vi "ApplyTableAppearance_benchmarking.vi"(6 "Defer Updates? (T)":bool=TRUE, 7 "Layout Ring Ref":refnum<vi>, 8 "error in (no error)":errorcluster, 9 "Mode Index":i32=2, 10 "Col Array in":refnum<class "Column.lvclass">[](array[class]), 11 "Table Ref in":refnum<vi>) -> (0 "error out":errorcluster, 3 "Table Ref out":refnum<vi>)   [LabVIEW 2013]
doc: "(Re)Initialize table appearance from column (appearance) array. A layout reference is required so that the existing layout view is preserved. The user can choose not to 'defer panel updates,' although the default is recommended to keep the program responsive.\n\nThis VI is read-only w.r.t. the column array."
uses:
  ColumnVIs/Column/Column.lvclass
  <vilib>/Utility/miscctls.llb/LVRowAndColumnTypeDef.ctl
  Globals/StdRowHeightGlobal.vi
panel:
  out "UnDefer (ms)":u32
  out "Layout (ms)":u32
  out "Rows + Mode (ms)":u32
  out "InitAppear (ms)":u32
  out "Reset Table (ms)":u32
  out "Defer (ms)":u32
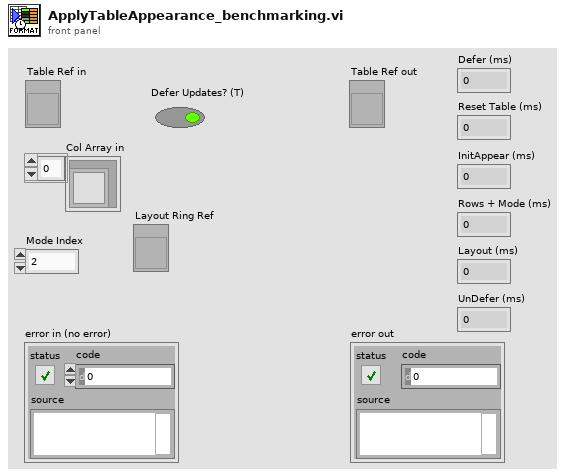
[diagram p1: front panel]
types:
  T1 = typedef "LVRowAndColumnTypeDef.ctl" = cluster{"Row":i32, "Column":i32}
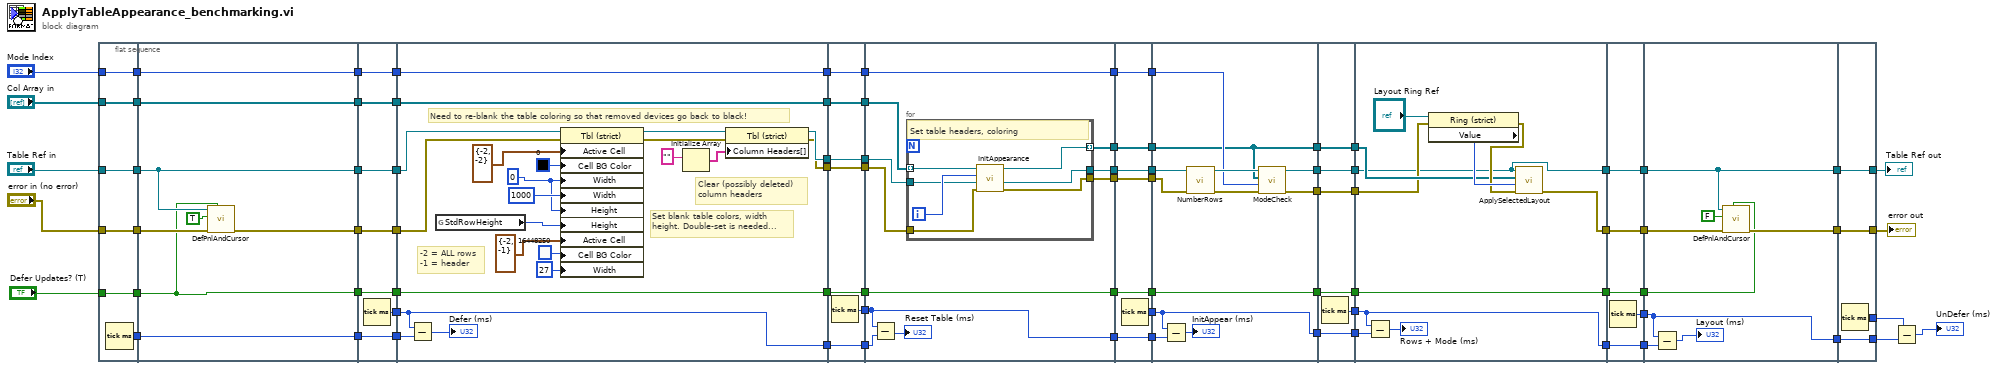
[diagram p0: block diagram]
diagram:
  n1 = flat-sequence {
    tunnel: "Mode Index" -> [w80]
    tunnel: "Col Array in" -> [w81]
    tunnel: "Table Ref in" -> [w82]
    tunnel: "Defer Updates? (T)" -> [w83]
    tunnel: "error in (no error)" -> [w84]
    tunnel: [w84] -> w70
    tunnel: [w83] -> w69
    tunnel: [w82] -> w68
    tunnel: [w81] -> w67
    tunnel: [w80] -> w66
    tunnel: [w79] -> w53
    tunnel: [w88] -> w65
    tunnel: [w87] -> w63
    tunnel: [w92] -> w61
    tunnel: [w91] -> w59
    tunnel: [w86] -> w57
    tunnel: w70 -> [w89]
    tunnel: w69 -> [w86]
    tunnel: w68 -> [w87]
    tunnel: w67 -> [w92]
    tunnel: w66 -> [w91]
    tunnel: [w90] -> w54
    tunnel: w53 -> [w90]
    tunnel: w65 -> [w99]
    tunnel: [w99] -> w64
    tunnel: w63 -> [w98]
    tunnel: [w98] -> w62
    tunnel: w61 -> [w97]
    tunnel: [w97] -> w60
    tunnel: w59 -> [w96]
    tunnel: [w96] -> w58
    tunnel: w57 -> [w95]
    tunnel: [w95] -> w56
    tunnel: [w94] -> w55
    tunnel: w54 -> [w94]
    tunnel: [w93] -> w52
    tunnel: w64 -> [w110]
    tunnel: w62 -> [w109]
    tunnel: w60 -> [w121]
    tunnel: w58 -> [w120]
    tunnel: [w111] -> w51
    tunnel: [w121] -> w49
    tunnel: [w120] -> w47
    tunnel: [w112] -> w45
    tunnel: w56 -> [w112]
    tunnel: [w108] -> w43
    tunnel: w55 -> [w106]
    tunnel: w52 -> [w105]
    tunnel: [w105] -> w40
    tunnel: w51 -> [w128]
    tunnel: [w128] -> w50
    tunnel: w49 -> [w127]
    tunnel: [w127] -> w48
    tunnel: w47 -> [w126]
    tunnel: [w126] -> w46
    tunnel: w45 -> [w125]
    tunnel: [w125] -> w44
    tunnel: w43 -> [w124]
    tunnel: [w124] -> w42
    tunnel: [w123] -> w41
    tunnel: w40 -> [w123]
    tunnel: [w122] -> w39
    tunnel: w50 -> [w133]
    tunnel: w48 -> [w138]
    tunnel: w46 -> [w139]
    tunnel: [w135] -> w38
    tunnel: [w139] -> w36
    tunnel: [w137] -> w34
    tunnel: [w136] -> w32
    tunnel: w44 -> [w136]
    tunnel: [w134] -> w30
    tunnel: w42 -> [w132]
    tunnel: w41 -> [w130]
    tunnel: w39 -> [w129]
    tunnel: [w129] -> w27
    tunnel: w38 -> [w153]
    tunnel: [w153] -> w37
    tunnel: w36 -> [w152]
    tunnel: [w152] -> w35
    tunnel: w34 -> [w151]
    tunnel: [w151] -> w33
    tunnel: w32 -> [w150]
    tunnel: [w150] -> w31
    tunnel: w30 -> [w149]
    tunnel: [w149] -> w29
    tunnel: [w148] -> w28
    tunnel: w27 -> [w148]
    tunnel: [w147] -> w26
    tunnel: w37 -> [w159]
    tunnel: w35 -> [w163]
    tunnel: [w158] -> w25
    tunnel: w33 -> [w162]
    tunnel: [w162] -> w23
    tunnel: w31 -> [w161]
    tunnel: [w161] -> w21
    tunnel: [w160] -> w19
    tunnel: w29 -> [w157]
    tunnel: w28 -> [w155]
    tunnel: w26 -> [w154]
    tunnel: [w154] -> w15
    tunnel: w25 -> [w171]
    tunnel: [w171] -> w24
    tunnel: w23 -> [w170]
    tunnel: [w170] -> w22
    tunnel: w21 -> [w169]
    tunnel: [w169] -> w20
    tunnel: w19 -> [w168]
    tunnel: [w168] -> w18
    tunnel: [w167] -> w17
    tunnel: [w166] -> w16
    tunnel: w15 -> [w166]
    tunnel: w24 -> [w175]
    tunnel: [w177] -> w14
    tunnel: [w175] -> w12
    tunnel: w22 -> [w179]
    tunnel: [w178] -> w10
    tunnel: w20 -> [w178]
    tunnel: w18 -> [w176]
    tunnel: w17 -> [w172]
    tunnel: w16 -> [w173]
    tunnel: [w172] -> w6
    tunnel: w14 -> [w187]
    tunnel: [w187] -> w13
    tunnel: w12 -> [w186]
    tunnel: [w186] -> w11
    tunnel: w10 -> [w185]
    tunnel: [w185] -> w9
    tunnel: [w184] -> w8
    tunnel: [w183] -> w7
    tunnel: w6 -> [w183]
    tunnel: w13 -> [w192]
    tunnel: w11 -> [w189]
    tunnel: w9 -> [w188]
    tunnel: w8 -> [w193]
    tunnel: w7 -> [w194]
    tunnel: [w191] -> w5
    tunnel: [w189] -> w4
    tunnel: [w193] -> w2
    tunnel: [w198] -> w73
    tunnel: [w199] -> w72
    tunnel: w5 -> [w199]
    tunnel: w4 -> [w198]
    tunnel: [w197] -> w3
    tunnel: w2 -> [w196]
    tunnel: [w196] -> w1
    frame #0 {
      n2 = Tick Count (ms)() -> (millisecond timer value=w79:u32)
    }
    frame #1 {
      n3 = call "DefPnlAndCursor.vi"("AllowDefPan? (T)"=w86, "error in (no error)"=w89, "DeferPanUpdts?"=TRUE, "Tbl Ctrl Refnum"=w87) -> ("error out"=w88:errorcluster)  [unwired: 7 in]
    }
    frame #2 {
      n4 = Tick Count (ms)() -> (millisecond timer value=w93:u32)
    }
    frame #3 {
      w101 = u32 0 ("Active Cell:Cell Size:Height")
      # "Clear (possibly deleted)\ncolumn headers"
      # "Need to re-blank the table coloring so that removed devices go back to black!"
      # "-2 = ALL rows\n-1 = header"
      # "Set blank table colors, width\nheight. Double-set is needed..."
      n5 = Subtract(x=w105, y=w106) -> (x-y=→"Defer (ms)":u32)
      n6 = global read "StdRowHeightGlobal.vi" "StdRowHeight"() -> (w102:u32)
      n7 = property class="Tbl (strict)"(reference=w109, error in=w110, "Active Cell"=T1 {"Row"=-2, "Column"=-2} ("RowAndCollumn"), "Cell BG Color"=u32 0, "Width"=w101, "Width"=u32 1000 ("Active Cell:Cell Size:Width"), "Height"=w101, "Height"=w102, "Active Cell"=T1 {"Row"=-2, "Column"=-1} ("RowAndCollumn"), "Cell BG Color"=u32 16448250, "Width"=u32 27 ("Active Cell:Cell Size:Width")) -> (reference out=w116:refnum<vi>, error out=w117:errorcluster)
      n8 = Initialize Array("") -> (w119:string[])  [unwired: 1 in]
      n9 = property class="Tbl (strict)"(reference=w116, error in=w117, "Column Headers[]"=w119) -> (reference out=w111:refnum<vi>, error out=w108:errorcluster)
    }
    frame #4 {
      n10 = Tick Count (ms)() -> (millisecond timer value=w122:u32)
    }
    frame #5 {
      n11 = Subtract(x=w129, y=w130) -> (x-y=→"Reset Table (ms)":u32)
      n12 = for {
        tunnel: [w146] -> w134
        tunnel: [w145] -> w135
        tunnel: [w143] -> w137 mode=indexing
        tunnel: w138 -> [w142] mode=indexing
        tunnel: w133 -> [w141]
        tunnel: w132 -> [w140]
        i -> [w144]
        # "Set table headers, coloring"
        n13 = call-dynamic "InitAppearance.vi"("error in (no error)"=w140, "Table Ref in"=w141, "Col #"=w144, "Column in"=w142) -> ("error out"=w146:errorcluster, "Table Ref out"=w145:refnum<vi>, "Column out"=w143:refnum<class "Column.lvclass">)  [unwired: 5 in]
      }
    }
    frame #6 {
      n14 = Tick Count (ms)() -> (millisecond timer value=w147:u32)
    }
    frame #7 {
      n15 = Subtract(x=w154, y=w155) -> (x-y=→"InitAppear (ms)":u32)
      n16 = call "NumberRows.vi"("error in (no error)"=w157, "Table Ref in"=w159) -> ("error out"=w164:errorcluster, "Table Ref out"=w165:refnum<vi>)  [unwired: 8 in]
      n17 = call "ModeCheck.vi"("error in (no error)"=w164, "mode col. index"=w163, "Col Array in"=w162, "Table Ref in"=w165) -> ("error out"=w160:errorcluster, "Table Ref out"=w158:refnum<vi>)  [unwired: 6 in]
    }
    frame #8 {
      n18 = Tick Count (ms)() -> (millisecond timer value=w167:u32)
    }
    frame #9 {
      n19 = Subtract(x=w172, y=w173) -> (x-y=→"Rows + Mode (ms)":u32)
      n20 = property class="Ring (strict)"(reference="Layout Ring Ref", error in=w176) -> (error out=w181:errorcluster, "Value"=w182:i32)  [unwired: 1 out]
      n21 = call "ApplySelectedLayout.vi"("error in (no error)"=w181, "Layout index"=w182, "Col array"=w179, "Tbl Refnum"=w175) -> ("error out"=w177:errorcluster)  [unwired: 7 in]
    }
    frame #10 {
      n22 = Tick Count (ms)() -> (millisecond timer value=w184:u32)
    }
    frame #11 {
      n23 = Subtract(x=w193, y=w194) -> (x-y=→"Layout (ms)":u32)
      n24 = call "DefPnlAndCursor.vi"("AllowDefPan? (T)"=w188, "error in (no error)"=w192, "DeferPanUpdts?"=FALSE, "Tbl Ctrl Refnum"=w189) -> ("error out"=w191:errorcluster)  [unwired: 7 in]
    }
    frame #12 {
      n25 = Tick Count (ms)() -> (millisecond timer value=w197:u32)
    }
  }
  n26 = Subtract(x=w3, y=w1) -> (x-y=→"UnDefer (ms)":u32)
  "error out" <- w72
  "Table Ref out" <- w73
